vi "Get Column Names.vi"(8 "error in (no error)":errorcluster, 11 "SQL Statement in":refnum<class "SQL Statement.lvclass">) -> (0 "error out":errorcluster, 2 "Column Names":string[](array[string]), 3 "SQL Statement out":refnum<class "SQL Statement.lvclass">)   [LabVIEW 2023, in "SQLite.lvlib" / "SQL Statement.lvclass"]
doc: "Get the names of all the cloumns in the result set."
uses:
  SQL Statement.lvclass
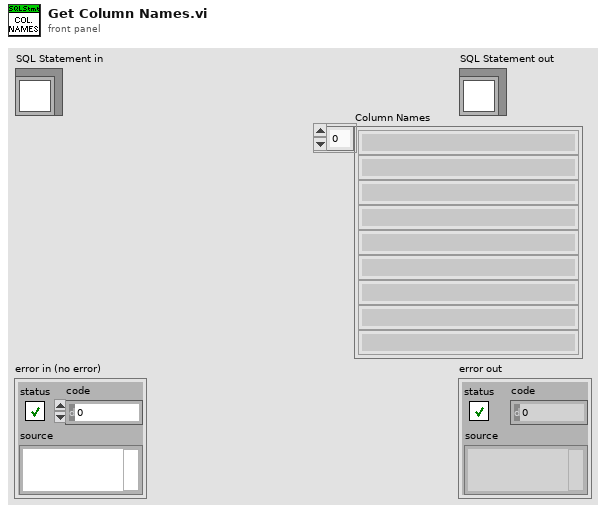
[diagram p1: front panel]
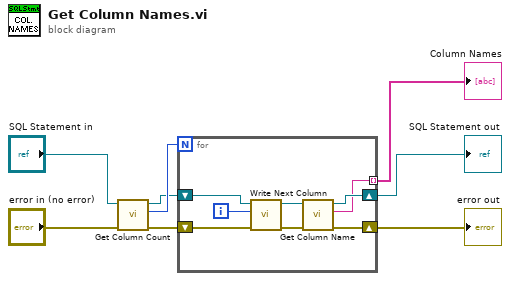
[diagram p0: block diagram]
diagram:
  n1 = call "Get Column Count.vi"("error in (no error)"="error in (no error)", "SQL Statement in"="SQL Statement in") -> ("error out"=w2:errorcluster, "Number of Columns"=w4:i32, "SQL Statement out"=w3:refnum<class "SQL Statement.lvclass">)  [unwired: 7 in]
  n2 = for {
    N: w4 -> [_]
    shift-right: [w10] -> w5
    shift-left: w3 -> [w16]
    shift-right: [w11] -> w7
    shift-left: w2 -> [w14]
    tunnel: [w9] -> w1 mode=indexing
    i -> [w15]
    n3 = call "Write Next Column.vi"("error in (no error)"=w14, "Next Column"=w15, "SQL Statement in"=w16) -> ("error out"=w12:errorcluster, "SQL Statement out"=w13:refnum<class "SQL Statement.lvclass">)  [unwired: 7 in]
    n4 = call "Get Column Name.vi"("error in (no error)"=w12, "SQL Statement in"=w13) -> ("error out"=w11:errorcluster, "Column Name"=w9:string, "SQL Statement out"=w10:refnum<class "SQL Statement.lvclass">)  [unwired: 7 in]
  }
  "error out" <- w7
  "SQL Statement out" <- w5
  "Column Names" <- w1
